vi "write_data.vi"(4 "Data":i16[](array[numeric]), 5 "Root Path":path, 6 "N Files In":i16, 7 "Bird Name":string, 8 "RefNum In":refnum<file>, 9 "File Open In":bool) -> (0 "N Files Out":i16, 1 "File Open Out":bool, 2 "Output File Path":path, 3 "RefNum Out":refnum<file>)   [LabVIEW 2018]
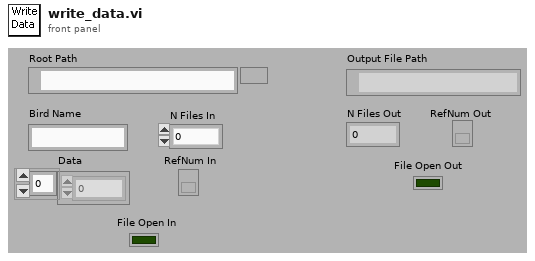
[diagram p1: front panel]
types:
  T1 = enum16{"open", "open or create", "create or replace", "create", "open (read only)"}
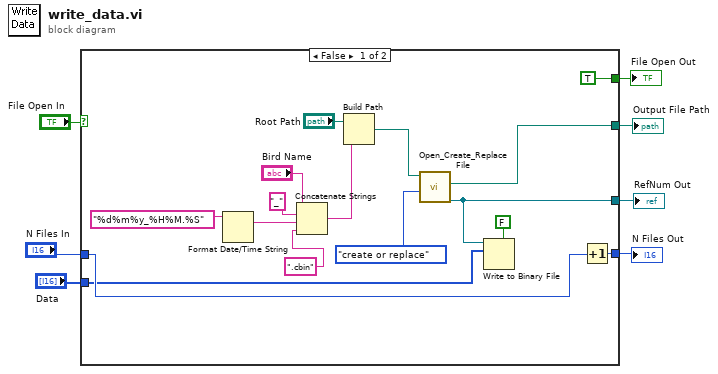
[diagram p0: block diagram]
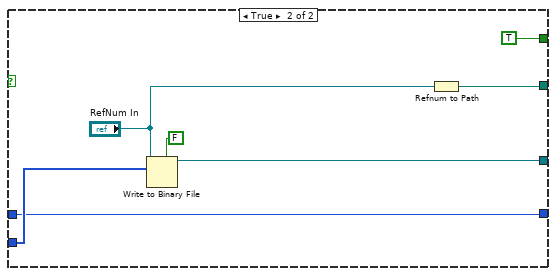
[diagram p2: hidden frame]
diagram:
  n1 = case shown="False" "File Open In" {
    tunnel: "Data" -> [w14 w30]
    tunnel: [w15 w29] -> w1
    tunnel: "N Files In" -> [w19 w28]
    tunnel: [w22 w28] -> w3
    tunnel: [w16 w27] -> w2
    tunnel: [TRUE TRUE] -> w6
    frame False {
      n2 = Format Date/Time String(time format string (%c)="%d%m%y_%H%M.%S") -> (date/time string=w20:string)  [unwired: 2 in]
      n3 = Concatenate Strings("Bird Name", "_" ("Substring"), w20, ".cbin" ("Substring")) -> (w18:string)
      n4 = Build Path(base path="Root Path", name or relative path=w18) -> (appended path=w17:path)
      n5 = call <vilib>:"Open_Create_Replace File.vi"("function (open:0)"=T1."create or replace", "file path"=w17) -> ("new file path"=w16:path, "refnum"=w15:refnum<file>)  [unwired: 6 in, 2 out]
      n6 = Write to Binary File(file (use dialog)=w15, data=w14, 5:FALSE ("prepend array or string size? (T)")) -> ()  [unwired: 3 in, 3 out]
      n7 = Increment(x=w19) -> (x+1=w22:i16)
    }
    frame True {
      n8 = Write to Binary File(file (use dialog)="RefNum In", data=w30, 5:FALSE ("prepend array or string size? (T)")) -> (refnum out=w29:refnum<file>)  [unwired: 3 in, 2 out]
      n9 = Refnum to Path(1:"RefNum In") -> (0:w27:path)
    }
  }
  "File Open Out" <- w6
  "N Files Out" <- w3
  "Output File Path" <- w2
  "RefNum Out" <- w1
